vi "FTW-Container-Array-Build.vi"(0 "FTW-Container In":refnum<class "FTW-Container.lvclass">, 7 "Array Elements":refnum<class "FTW-Container.lvclass">[](array[class]), 11 "error in":errorcluster) -> (4 "FTW-Container Out":refnum<class "FTW-Container.lvclass">, 15 "error out":errorcluster)   [LabVIEW 2015, in "FTW-Container.lvclass"]
uses:
  FTW-Container.lvclass
  FTW-Container.lvclass/FTW-Container.ctl
  <vilib>/Utility/Data Type/NI_Data Type.lvlib
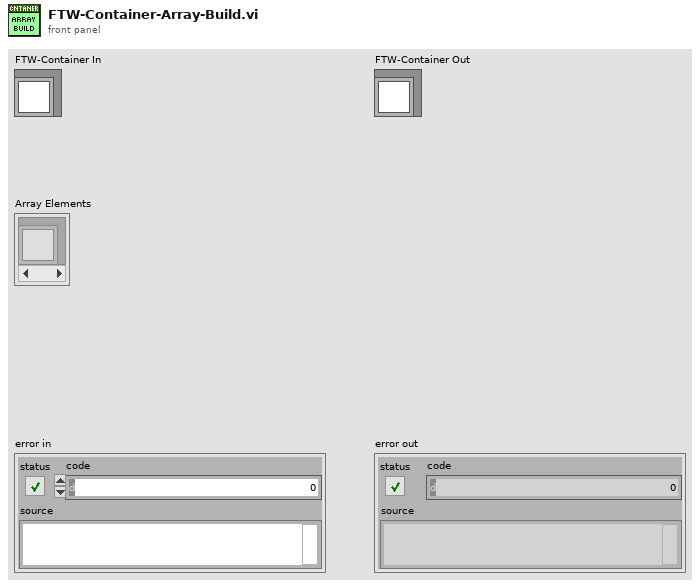
[diagram p1: front panel]
types:
  T1 = typedef "NI_Data Type.lvlib/Data Type.ctl" = enum8{"Invalid Type", "Void", "I8", "I16", "I32", "I64", "U8", "U16", "U32", "U64", "Single Float", "Double Float", "Extended Float", "Single Complex", "Double Complex", "Extended Complex", "Enum U8", "Enum U16", "Enum U32", "Enum U64", "Single Float With Unit", "Double Float With Unit", "Extended Float With Unit", "Single Complex with Unit", "Double Complex with Unit", "Extended Complex with Unit", "Boolean", "String", "Path", "Picture", "Tag", "Array", "Cluster", "Variant", "LV Variant", "Waveform", "Timestamp", "Digital Waveform", "Digital Data", "ExpressData", "Refnum", "External Data", "VI", "Poly VI", "LabVIEW Class Instance", "Fixed Point"}
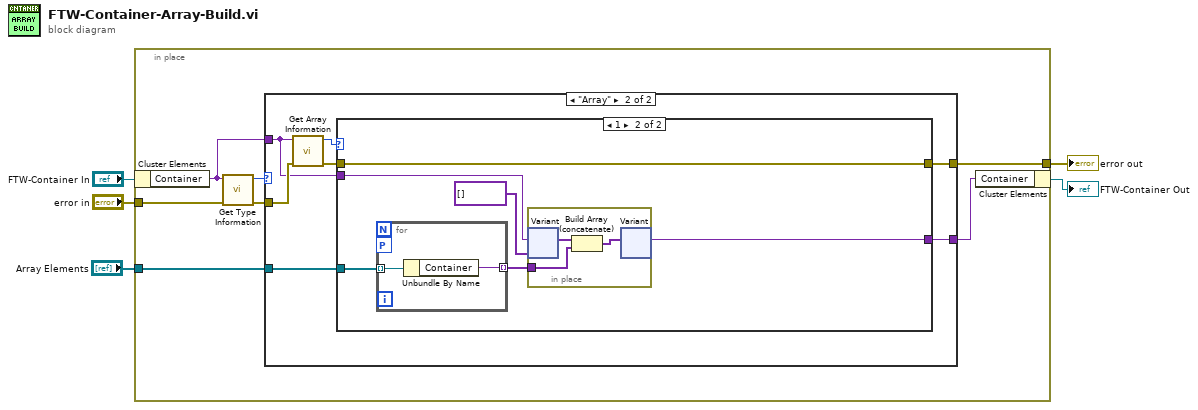
[diagram p0: block diagram]
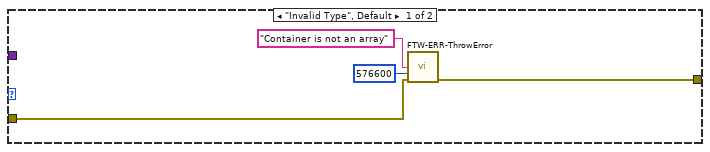
[diagram p2: hidden frame]
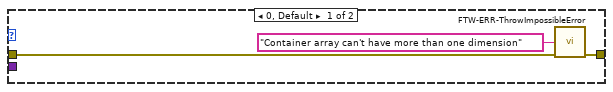
[diagram p3: hidden frame]
diagram:
  n1 = in-place {
    in-place-border: "error in" -> [w12]
    in-place-border: [w10] -> w4
    in-place-border: "Array Elements" -> [w8]
    n2 = in-place-cluster #1("FTW-Container In") -> ("Container"=w7:variant)
    n3 = call <vilib>:"Get Type Information.vi"("error in (no error)"=w12, "Variant"=w7) -> ("error out"=w11:errorcluster, "Type"=w9:T1)  [unwired: 5 in, 3 out]
    n4 = case shown="\"Array\"" w9 {
      tunnel: w11 -> [w16 w21]
      tunnel: [w15 w20] -> w10
      tunnel: w7 -> [_ w19]
      tunnel: w8 -> [_ w18]
      tunnel: [_ w17] -> w6
      frame "Invalid Type", Default {
        n5 = call "FTW-ERR-ThrowError.vi"("Error Message"="Container is not an array", "Error Code"=576600, "error in"=w16) -> ("error out"=w15:errorcluster)  [unwired: 12 in]
      }
      frame "Array" {
        n6 = call <vilib>:"Get Array Information.vi"("error in (no error)"=w21, "Variant"=w19) -> ("error out"=w23:errorcluster, "Number of Dimensions"=w22:i32)  [unwired: 6 in, 2 out]
        n7 = case shown="1" w22 {
          tunnel: w23 -> [w26 w32]
          tunnel: w19 -> [_ w31]
          tunnel: [w25 w32] -> w20
          tunnel: w18 -> [_ w29]
          tunnel: [_ w27] -> w17
          frame 0, Default {
            n8 = call "FTW-ERR-ThrowImpossibleError.vi"("Reason this error should never happen"="Container array can't have more than one dimension", "error in"=w26) -> ("error out"=w25:errorcluster)  [unwired: 13 in]
          }
          frame 1 {
            n9 = for {
              tunnel: w29 -> [w34] mode=indexing
              tunnel: [w33] -> w28 mode=indexing
              workers-P: _ -> [_]
              n10 = Unbundle By Name(w34) -> ("Container"=w33:variant)
            }
            n11 = in-place {
              in-place-border: w28 -> [w35]
              n12 = in-place-variant #2(w31, variant[] []) -> (w37:variant[])  [unwired: 1 out]
              n13 = Build Array (concatenate)(w37, w35) -> (w36:variant[])
              n14 = in-place-variant #2(w36) -> (w27:variant)  [unwired: 1 out]
            }
          }
        }
      }
    }
    n15 = in-place-cluster #1("Container"=w6) -> (→"FTW-Container Out":refnum<class "FTW-Container.lvclass">)
  }
  "error out" <- w4
